vi "rs3 create device2.vi"(8 "error in (no error)":errorcluster, 10 "Device index":i32, 11 "device list in":u64) -> (0 "error out":errorcluster, 1 "Dev out":u64, 2 "error":u64, 3 "device list out":u64)   [LabVIEW 2017, in "libRealSense3.lvlib"]
doc: "Creates a DEVICE from a specific Device list and DEVICE INDEX.\n\nINPUT: \nDevice Index Select the device. Device=0 is normally a RealSense device. Device=1 is often PC camera.\nDevice list Input Handle of device list\n\nOUTPUT:\nDev out This is the DEVICE handle\nError Error=0 is no error"
uses:
  libRealSense3.lvlib
  realsense2.dll
panel:
  # "RS3 Create Device"
  # "(C) 2017 Intel Corp.,  AGJ"
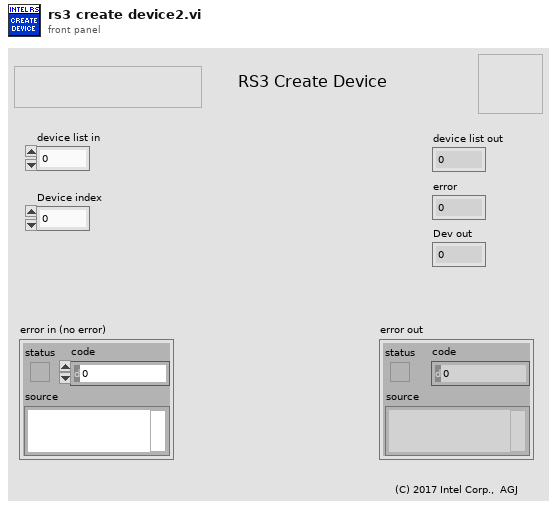
[diagram p1: front panel]
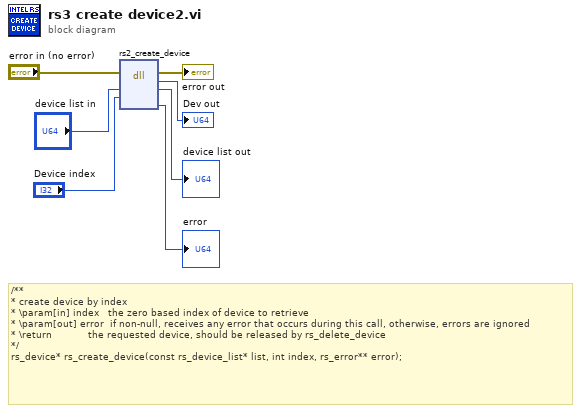
[diagram p0: block diagram]
diagram:
  # "/**\n* create device by index\n* \\param[in] index   the zero based index of device to retrieve\n* \\param[out] error  if non-null, receives any error that occurs during this call, otherwise, errors are ignored\n* \\return            the requested device, should be released by rs_delete_device\n*/\nrs_device* rs_create_device(const rs_device_list* list, int index, rs_error** error);"
  n1 = dll-call lib="C:/Users/smartek/Desktop/labview/realsense2.dll" fn="rs2_create_device"(error in="error in (no error)", "device list"="device list in", "index"="Device index") -> (error out=→"error out":errorcluster, "device"=→"Dev out":u64, "device list"=→"device list out":u64, "error"=→"error":u64)  [unwired: 4 in, 1 out]
